vi "Speed Mode.vi"(8 "error in (no error)":errorcluster, 10 "String":string, 11 "Speed Mode in":refnum<class "Speed Mode.lvclass">) -> (0 "error out":errorcluster, 2 "This VI":refnum<vi>, 3 "Speed Mode out":refnum<class "Speed Mode.lvclass">)   [LabVIEW 2020, in "Speed Mode.lvclass"]
uses:
  Speed Mode.lvclass
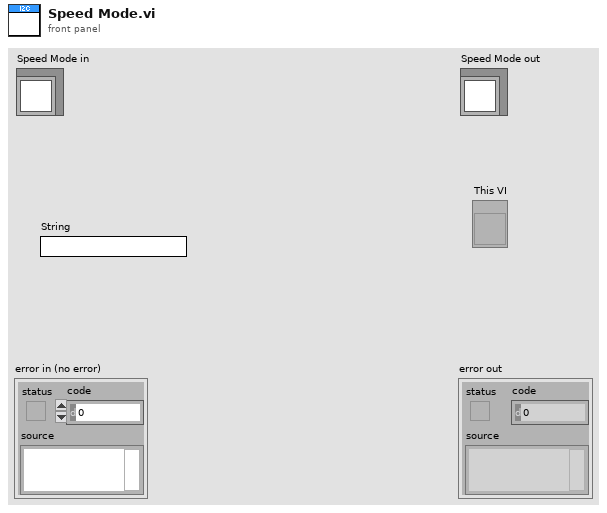
[diagram p1: front panel]
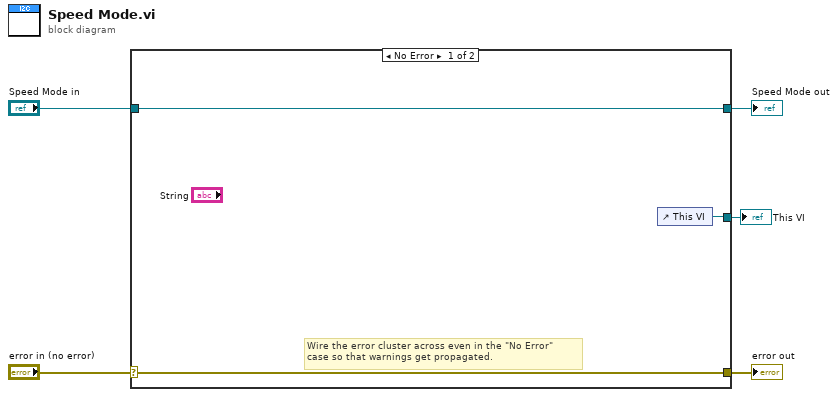
[diagram p0: block diagram]
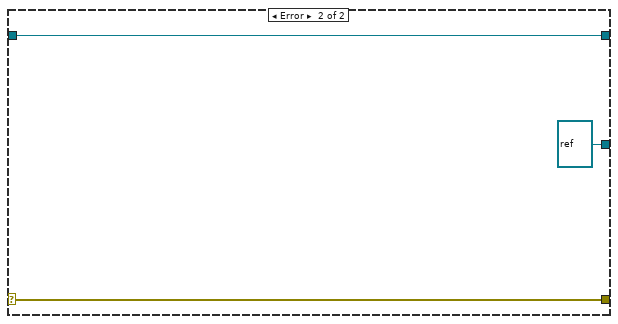
[diagram p2: hidden frame]
diagram:
  n1 = case shown="No Error" "error in (no error)" {
    selector: "error in (no error)" -> [w7 w11]
    tunnel: [w7 w11] -> w4
    tunnel: [w8 w10] -> w2
    tunnel: "Speed Mode in" -> [w8 w10]
    tunnel: [w6 refnum<vi> refnum ("This VI")] -> w1
    frame No Error {
      # "Wire the error cluster across even in the \"No Error\"\ncase so that warnings get propagated."
      n2 = control-ref of="This VI"() -> (w6:refnum<vi>)
    }
    frame Error {
    }
  }
  "error out" <- w4
  "Speed Mode out" <- w2
  "This VI" <- w1
